vi "Request Value Reference Updates.vi"(7 "Return Error If Unwritten? (T)":bool=TRUE, 8 "error in (no error)":errorcluster, 9 "Datum Type/Initial Value":variant, 10 "Datum Name":string, 11 "IObserver in":refnum<class "IObserver.lvclass">) -> (0 "error out":errorcluster, 1 "ValueReferenceTransport":refnum<class "ValueReferenceTransport.lvclass">, 2 "Subscription Policy":T1, 3 "IObserver out":refnum<class "IObserver.lvclass">)   [LabVIEW 2018, in "MVA Framework.lvlib" / "IObserver.lvlib" / "IObserver.lvclass"]
doc: "请求值引用更新"
uses:
  IObserver.lvclass
  IMediator/SubscriptionRequest/SubscriptionRequest.lvclass
  <vilib>/ActorFramework/Actor/Actor.lvclass
  IMediator/ISubscriptionPolicy/ISubscriptionPolicy.lvclass
  SubscriptionPolicy/ValueChangeSubscription/ValueChangeSubscription.lvclass
  IObserver Messages/Subscribe Msg/Subscribe Msg.lvclass
  composed-transport/Source/Concrete/ValueReferenceTransport/ValueReferenceTransport.lvclass
  C:/Program Files/National Instruments/LabVIEW 2020/vi.lib/ActorFramework/Actor/Actor.lvclass
  IMediator/ISubscriptionPolicy/ISubscriptionPolicy Reference.ctl
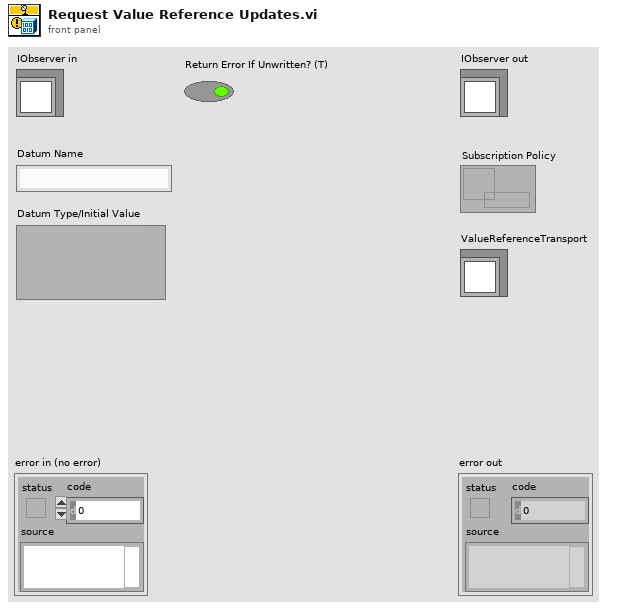
[diagram p1: front panel]
types:
  T1 = typedef "MVA Framework.lvlib/IMediator.lvlib/ISubscriptionPolicy.lvclass/ISubscriptionPolicy Reference.ctl" = refnum<data-value>
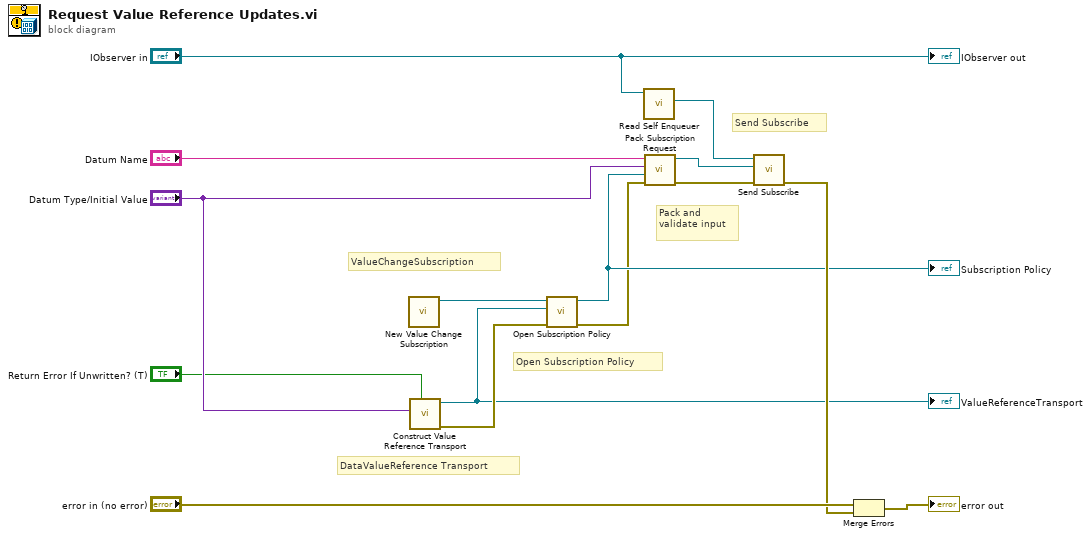
[diagram p0: block diagram]
diagram:
  # "ValueChangeSubscription"
  # "Open Subscription Policy"
  # "Send Subscribe"
  # "Pack and\nvalidate input"
  # "DataValueReference Transport"
  n1 = call "New Value Change Subscription.vi"() -> ("ValueChangeSubscription Out"=w13:refnum<class "ValueChangeSubscription.lvclass">)  [unwired: 11 in]
  n2 = call "Construct Value Reference Transport.vi"("Return Error If Unwritten? (T)"="Return Error If Unwritten? (T)", "Initial Value"="Datum Type/Initial Value") -> ("error out"=w7:errorcluster, "ValueReferenceTransport"=w4:refnum<class "ValueReferenceTransport.lvclass">)  [unwired: 8 in]
  "ValueReferenceTransport" <- w4
  n3 = call "Open Subscription Policy.vi"("error in (no error)"=w7, "Transport"=w4, "SubscriptionPolicy"=w13) -> ("error out"=w2:errorcluster, "Subscription Policy"=w6:T1)  [unwired: 7 in]
  "Subscription Policy" <- w6
  n4 = call <vilib>:"Read Self Enqueuer.vi"("Actor"="IObserver in") -> ("Self Enqueuer"=w8:refnum<class "Message Enqueuer.lvclass">)  [unwired: 10 in]
  n5 = call "Pack Subscription Request.vi"("error in (no error)"=w2, "Subscription Policy"=w6, "Type"="Datum Type/Initial Value", "Datum Name"="Datum Name") -> ("error out"=w1:errorcluster, "SubscriptionRequest"=w10:refnum<class "SubscriptionRequest.lvclass">)  [unwired: 6 in]
  n6 = call "Send Subscribe.vi"("error in (no error)"=w1, "SubscriptionRequest"=w10, "Message Enqueuer"=w8) -> ("error out"=w9:errorcluster)  [unwired: 7 in, 1 out]
  n7 = Merge Errors("error in (no error)", w9) -> (→"error out":errorcluster)
  "IObserver out" <- "IObserver in"
